vi "Write Source Path or URL.vi"(8 "error in (no error)":errorcluster, 10 "Source Path or URL":string, 11 "JSON Deserializer in":refnum<class "JSON Deserializer.lvclass">) -> (0 "error out":errorcluster, 3 "JSON Deserializer out":refnum<class "JSON Deserializer.lvclass">)   [LabVIEW 2020, in "JKI JSON Serialization.lvlib" / "JSON Deserializer.lvclass"]
uses:
  JSON Deserializer.lvclass
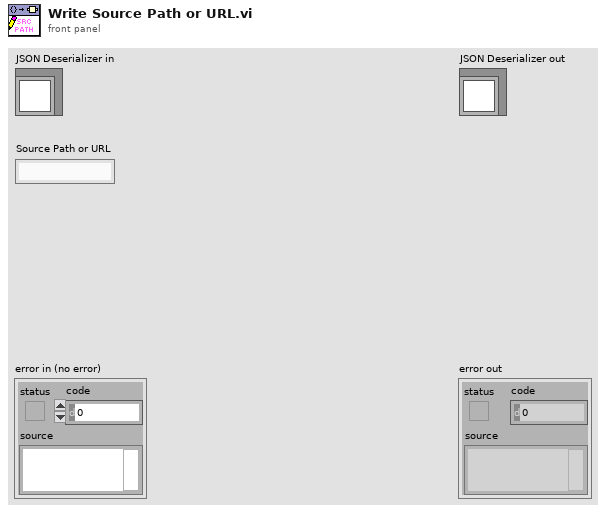
[diagram p1: front panel]
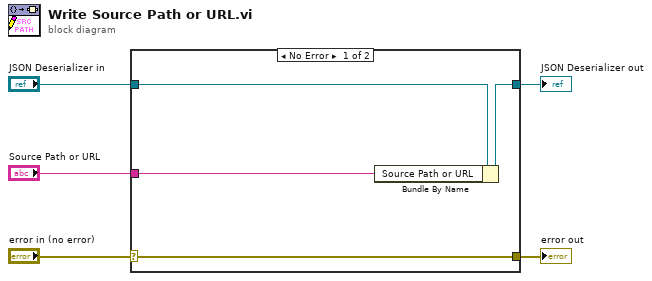
[diagram p0: block diagram]
diagram:
  n1 = case shown="No Error" "error in (no error)" {
    selector: "error in (no error)" -> [w9 w10]
    tunnel: [w9 w10] -> w4
    tunnel: [w7 w11] -> w2
    tunnel: "JSON Deserializer in" -> [w8 w11]
    tunnel: "Source Path or URL" -> [w6 _]
    frame No Error {
      n2 = Bundle By Name(cluster=w8, "Source Path or URL"=w6) -> (w7:refnum<class "JSON Deserializer.lvclass">)
    }
    frame Error {
    }
  }
  "error out" <- w4
  "JSON Deserializer out" <- w2
